vi "Get Subtype Description.vi"(8 "error in (no error)":errorcluster, 11 "Window Action in":refnum<class "Window Action.lvclass">) -> (0 "error out":errorcluster, 2 "Subtype Description":string, 3 "Window Action out":refnum<class "Window Action.lvclass">)   [LabVIEW 2020, in "MacroAssert.lvlib" / "Window Action.lvclass"]
doc: "Gets the subtype description for <B>Step in</B>, which describes what the step's subtype does specifically."
uses:
  Window Action.lvclass
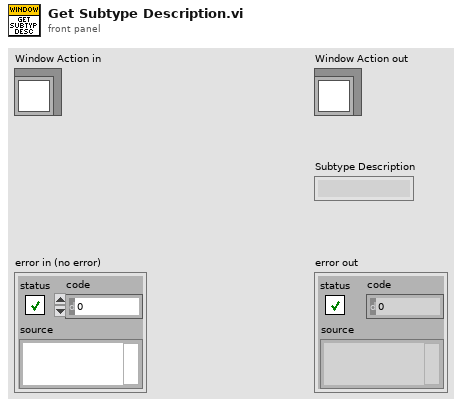
[diagram p1: front panel]
types:
  T1 = typedef "MacroAssert.lvlib/Window Action.lvclass/Window Action Type.ctl" = enum16{"Maximize Window", "Restore Window", "Minimize Window", "Close Window", "Bring Window to Front", "Send Window to Back"}
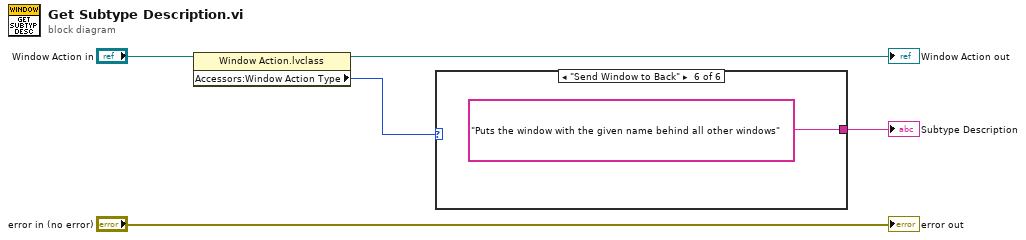
[diagram p0: block diagram]
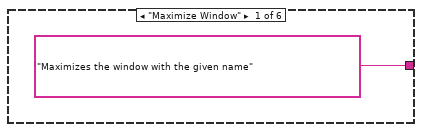
[diagram p2: hidden frame]
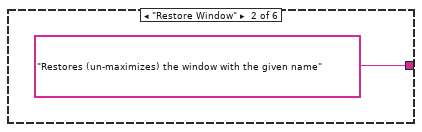
[diagram p3: hidden frame]
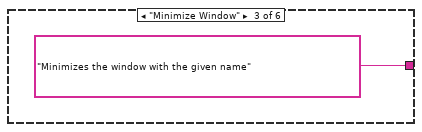
[diagram p4: hidden frame]
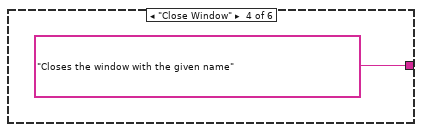
[diagram p5: hidden frame]
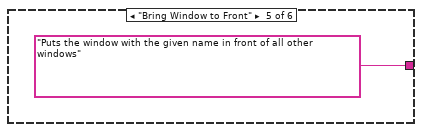
[diagram p6: hidden frame]
diagram:
  n1 = property class="Window Action.lvclass"(reference="Window Action in") -> (reference out=→"Window Action out":refnum<class "Window Action.lvclass">, "Accessors:Window Action Type"=w5:T1)  [unwired: 1 in, 1 out]
  n2 = case shown="\"Send Window to Back\"" w5 {
    tunnel: ["Maximizes the window with the given name" "Restores (un-maximizes) the window with the given name" "Minimizes the window with the given name" "Closes the window with the given name" "Puts the window with the given name in front of all other windows" "Puts the window with the given name behind all other windows"] -> w1
    frame "Maximize Window" {
    }
    frame "Restore Window" {
    }
    frame "Minimize Window" {
    }
    frame "Close Window" {
    }
    frame "Bring Window to Front" {
    }
    frame "Send Window to Back" {
    }
  }
  "Subtype Description" <- w1
  "error out" <- "error in (no error)"
